vi "Write json to PAR DB one.vi"(7 "conninfo":T1={"host"="localhost", "port"="5432", "client_encoding"="WIN1251", "dbname"="system", "user"="postgres", "password"=""}, 8 "error in (no error)":errorcluster, 10 "JSON Data In":string, 11 "PAR in":T2) -> (0 "error out":errorcluster, 3 "PAR out":T2)   [LabVIEW 2019, in "Inputs.lvlib"]
uses:
  Inputs.lvlib
  Ctl/Param.ctl
  Database/ctl/Coninfo.ctl
  Database/PostgreSQL2LabVIEW/libpqUtility64/src/PQexecute.vi
  Database/PostgreSQL2LabVIEW/libpqUtility64/src/PQconnect.vi
  Database/PostgreSQL2LabVIEW/libpqUtility64/src/PQclose.vi
  <vilib>/JDP Science/JSONtext/Find Multiple Items.vi
  Database/PostgreSQL2LabVIEW/libpqlv64/src/PQresultErrorMessage.vi
  Database/PostgreSQL2LabVIEW/libpqUtility64/src/PQclear.vi
  Database/PostgreSQL2LabVIEW/libpqlv64/src/PQsendQuery.vi
  Database/PostgreSQL2LabVIEW/libpqlv64/src/PQgetResult.vi
  Database/PostgreSQL2LabVIEW/libpqlv64/src/PQresultStatus.vi
  Database/PostgreSQL2LabVIEW/libpqlv64/src/PQfinish.vi
  Database/PostgreSQL2LabVIEW/libpqlv64/src/PQconnectdb.vi
  Database/PostgreSQL2LabVIEW/libpqlv64/src/PQerrorMessage.vi
  Database/PostgreSQL2LabVIEW/libpqlv64/src/PQstatus.vi
  <vilib>/dlg_ctls.llb/Space Constant.vi
  <vilib>/JDP Science/JSONtext/String Subset.vi
  <vilib>/JDP Science/JSONtext/support/Strip Quotes and Unescape.vi
  Database/PostgreSQL2LabVIEW/libpqlv64/src/PQclear.vi
  <vilib>/JDP Science/JSONtext/Parsing/Parse Full Path or Item Name.vi
  <vilib>/JDP Science/JSONtext/Offset/Find Item Locations by Path.vi
  <vilib>/JDP Science/JSONtext/support/Unescape JSON string.vi
  <vilib>/JDP Science/JSONtext/Get Array Elements.vi
  Userlib.lvlib
  Database/PostgreSQL.lvlib
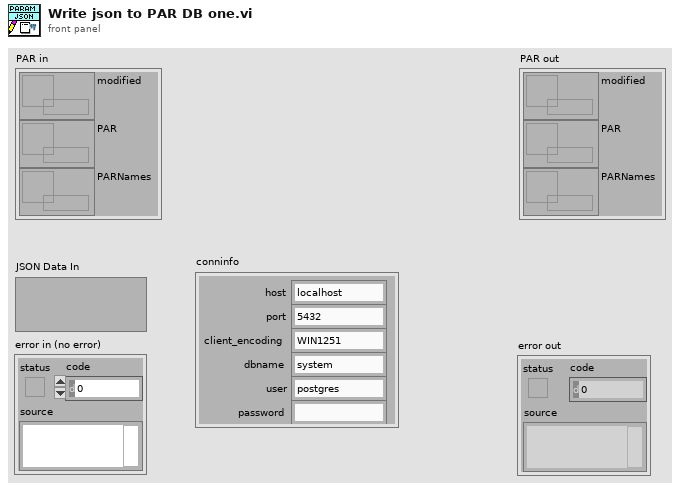
[diagram p1: front panel]
types:
  T1 = typedef "PostgreSQL.lvlib/Coninfo.ctl" = cluster{"host":string, "port":string, "client_encoding":string, "dbname":string, "user":string, "password":string}
  T2 = typedef "Inputs.lvlib/Param.ctl" = cluster{"modified":refnum<data-value>, "PAR":refnum<data-value>, "PARNames":refnum<data-value>}
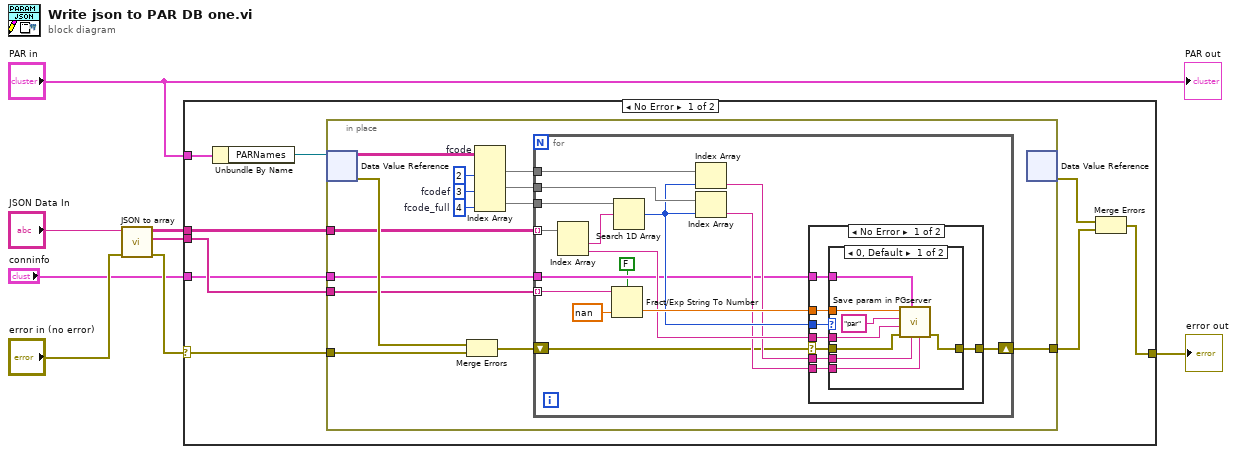
[diagram p0: block diagram]
diagram:
  n1 = call "JSON to array.vi"("error in (no error)"="error in (no error)", "JSON Data In"="JSON Data In") -> ("error out"=w5:errorcluster, "values"=w2:string[], "names"=w3:string[][])  [unwired: 7 in]
  n2 = case shown="No Error" w5 {
    selector: w5 -> [w10 w66]
    tunnel: [w16 w66] -> w8
    tunnel: "PAR in" -> [w17 _]
    tunnel: w2 -> [w15 _]
    tunnel: w3 -> [w12 _]
    tunnel: "conninfo" -> [w9 _]
    frame No Error {
      n3 = Unbundle By Name(w17) -> ("PARNames"=w14:refnum<data-value>)
      n4 = in-place {
        in-place-border: w15 -> [w27]
        in-place-border: [w28] -> w11
        in-place-border: w12 -> [w25]
        in-place-border: w10 -> [w19]
        in-place-border: w9 -> [w18]
        w22 = 3  # fcodef
        w23 = 2  # fcode
        w24 = 4  # fcode_full
        n5 = in-place-dvr #1(w14) -> (w31:string[][], w29:errorcluster)
        n6 = Merge Errors(w29, w19) -> (w26:errorcluster)
        n7 = Index Array(array=w31, index (col) #1=w23, index (col) #2=w22, index (col) #3=w24) -> (element #1=w30:string[], element #2=w20:string[], element #3=w21:string[])  [unwired: 3 in]
        n8 = for {
          tunnel: w30 -> [w39]
          tunnel: w27 -> [w46] mode=indexing
          shift-right: [w47] -> w28
          shift-left: w26 -> [w34]
          tunnel: w25 -> [w43] mode=indexing
          tunnel: w21 -> [w40]
          tunnel: w20 -> [w38]
          tunnel: w18 -> [w33]
          n9 = Index Array(array=w43) -> (element #1=w42:string, element #2=w41:string)  [unwired: 2 in]
          n10 = Fract/Exp String To Number(use system decimal point (T)=FALSE, string=w46, default (0 dbl)=nan ("default (0 DBL)")) -> (number=w45:dbl)  [unwired: 1 in, 1 out]
          n11 = Search 1D Array(1D array=w40, element=w42) -> (index of element=w37:i32)  [unwired: 1 in]
          n12 = Index Array(array=w39, index=w37) -> (element=w36:string)
          n13 = Index Array(array=w38, index=w37) -> (element=w35:string)
          n14 = case shown="No Error" w34 {
            selector: w34 -> [w49 w65]
            tunnel: w45 -> [w55 _]
            tunnel: w37 -> [w54 _]
            tunnel: [w50 w65] -> w47
            tunnel: w41 -> [w53 _]
            tunnel: w36 -> [w52 _]
            tunnel: w35 -> [w51 _]
            tunnel: w33 -> [w48 _]
            frame No Error {
              n15 = case shown="0, Default" w54 {
                tunnel: w55 -> [w62 _]
                tunnel: w53 -> [w61 _]
                tunnel: w52 -> [w60 _]
                tunnel: w51 -> [w59 _]
                tunnel: w49 -> [w58 w64]
                tunnel: [w57 w64] -> w50
                tunnel: w48 -> [w56 _]
                frame 0, Default {
                  n16 = call "Save param in PGserver.vi"("Param row name 2"=w59, "Param row name1"=w60, "conninfo"=w56, "error in (no error)"=w58, "Param column Name"=w61, "Param Table"="par", "Parameter"=w62) -> ("error out"=w57:errorcluster)  [unwired: 4 in]
                }
                frame -1 {
                }
              }
            }
            frame Error {
            }
          }
        }
        n17 = in-place-dvr #1() -> (w13:errorcluster)  [unwired: 1 in, 1 out]
      }
      n18 = Merge Errors(w13, w11) -> (w16:errorcluster)
    }
    frame Error {
    }
  }
  "error out" <- w8
  "PAR out" <- "PAR in"
